vi "RSZVB Configure Calibration Standard.vi"(0 "VISA session":refnum<visa-resource-name>, 1 "Max. Freq [Hz]":dbl format="%^.3e", 2 "Length [mm]":dbl format="%^.3e", 3 "Loss":dbl format="%^.3e", 4 "C0/L0 (0.0)":dbl format="%^.3e", 5 "C1/L1 (0.0)":dbl format="%^.3e", 7 "error in (no error)":errorcluster {"code" format="%.0x"}, 8 "Min. Freq [Hz]":dbl format="%^.3e", 9 "C2/L2 (0.0)":dbl format="%^.3e", 10 "Serial Number":string, 12 "Kit":string, 13 "C3/L3 (0.0)":dbl format="%^.3e", 14 "Standard (0: Through (MM))":u16(ring) items=["Through (MM)", "Through (FF)", "Through (MF)", "Line 1 (MM)", "Line 1 (FF)", "Line 1 (MF)", "Offset short (sexless)", "Offset short (M)", "Offset short (F)", "Attenuation (MM)", "Attenuation (FF)", "Attenuation (MF)", "Symm Network (MM)", "Symm Network (FF)", "Symm Network (MF)", "Open (M)", "Open (F)", "Short (M)", "Short (F)", "Reflect (M)", "Reflect (F)", "Match (M)", "Match (F)", "Sliding Match (M)", "Sliding Match (F)", "Line 2 (MM)", "Line 2 (FF)", "Line 2 (MF)", "Line 3 (MM)", "Line 3 (FF)", "Line 3 (MF)", "Offset short 2 (M)", "Offset short 2 (F)", "Offset short 3 (M)", "Offset short 3 (F)"], 16 "Connector Type (0: N 50 ohms Kit)":i32(ring) items=["N 50 ohms Kit", "N 75 ohms Kit", "SMA Kit", "PC 7 Kit", "PC 3.5 Kit", "Sexless Usr Conn 1", "Usr Conn 2", "2.92mm Kit"], 17 "Approximation (0: Open)":i32(ring) items=["Open", "Short"]) -> (20 "dup VISA session":refnum<visa-resource-name>, 27 "error out":errorcluster {"code" format="%.0x"})   [LabVIEW 2011]
doc: "This VI defines the parameters of a calibration standard <std_type> for a specified connector type <conn_type>. A particular physical standard can be selected by specifying the name of the calibration kit and its serial number.\n\nRemote-control command(s):\n[SENSe<Ch>:]CORRection:CKIT:<conn_type>:<std_type> '<Ckit_Name>','<Std_No>',<Min_Freq>,<Max_Freq>,<El_Length>,<Loss>,<C0> | <L0>,<C1> | <L1>,<C2> | <L2>,<C3> | <L3>, OPEN | SHORt"
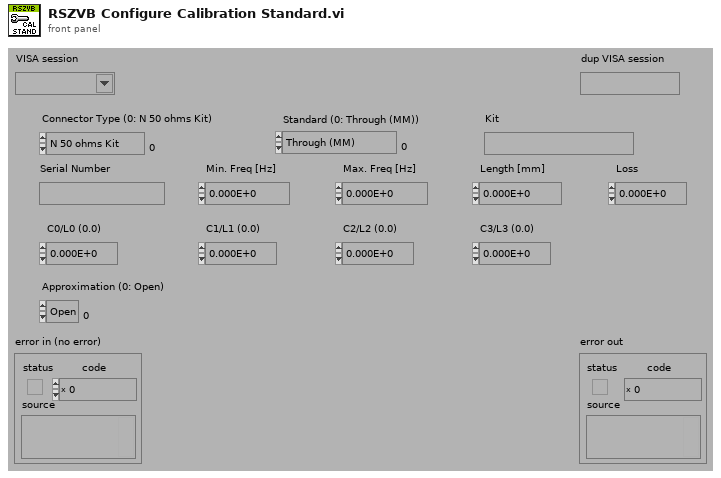
[diagram p1: front panel]
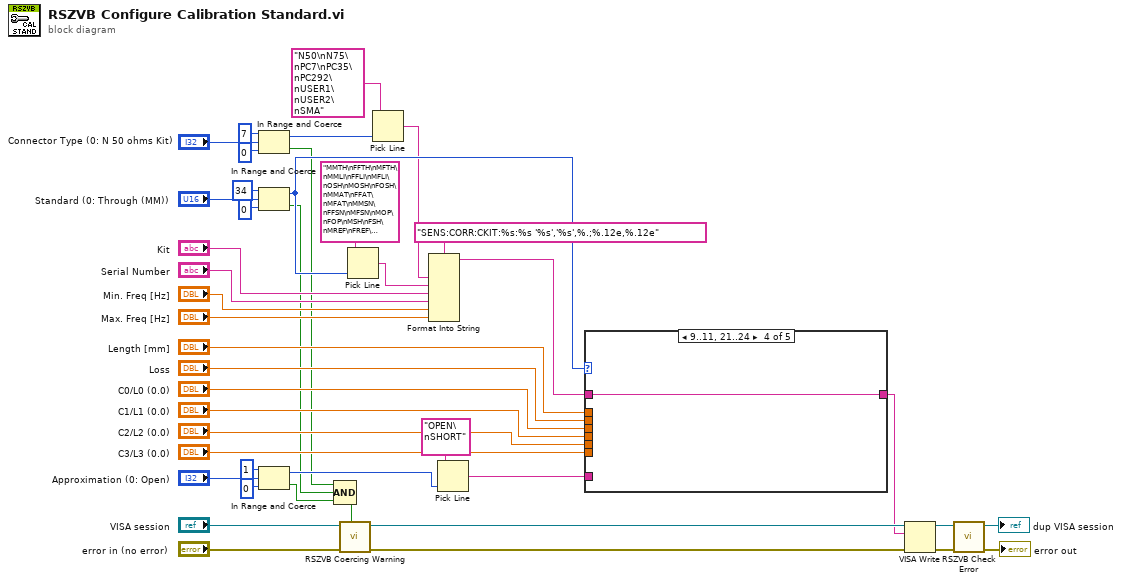
[diagram p0: block diagram]
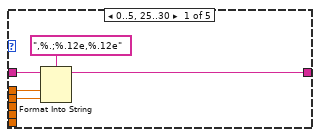
[diagram p2: hidden frame]
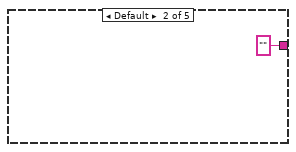
[diagram p3: hidden frame]
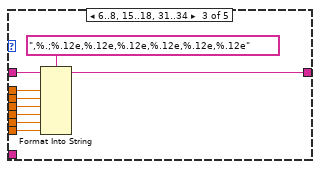
[diagram p4: hidden frame]
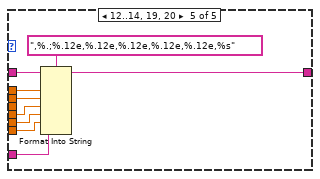
[diagram p5: hidden frame]
diagram:
  n1 = In Range and Coerce(upper limit=7 ("lower limit"), x="Connector Type (0: N 50 ohms Kit)", lower limit=0) -> (coerced(x)=w27:i32, In Range?=w2:bool)
  n2 = In Range and Coerce(upper limit=u16 34 ("lower limit"), x="Standard (0: Through (MM))", lower limit=u16 0) -> (coerced(x)=w13:u16, In Range?=w3:bool)
  n3 = In Range and Coerce(upper limit=1 ("lower limit"), x="Approximation (0: Open)", lower limit=0) -> (coerced(x)=w4:i32, In Range?=w18:bool)
  n4 = Compound Arithmetic op=AND(w2, w3, w18) -> (w17:bool)
  n5 = call "RSZVB Coercing Warning.vi"("In Range?"=w17, "error in (no error)"="error in (no error)", "VISA session"="VISA session") -> ("error out"=w42:errorcluster, "dup VISA session"=w43:refnum<visa-resource-name>)  [unwired: 7 in]
  n6 = Pick Line(multi-line string="MMTH\nFFTH\nMFTH\nMMLI\nFFLI\nMFLI\nOSH\nMOSH\nFOSH\nMMAT\nFFAT\nMFAT\nMMSN\nFFSN\nMFSN\nMOP\nFOP\nMSH\nFSH\nMREF\nFREF\nMMTC\nFMTC\nMSM\nFSM\nMMLI2\nFFLI2\nMFLI2\nMMLI3\nFFLI3\nMFLI3\nMOSHORT2\nFOSHORT2\nMOSHORT3\nFOSHORT3", line index=w13) -> (output string=w7:string)  [unwired: 1 in]
  n7 = Pick Line(multi-line string="N50\nN75\nPC7\nPC35\nPC292\nUSER1\nUSER2\nSMA", line index=w27) -> (output string=w6:string)  [unwired: 1 in]
  n8 = Format Into String(format string="SENS:CORR:CKIT:%s:%s '%s','%s',%.;%.12e,%.12e", w6, w7, "Kit", "Serial Number", "Min. Freq [Hz]", "Max. Freq [Hz]") -> (resulting string=w5:string)  [unwired: 2 in, 1 out]
  n9 = Pick Line(multi-line string="OPEN\nSHORT", line index=w4) -> (output string=w19:string)  [unwired: 1 in]
  n10 = case shown="9..11, 21..24" w13 {
    tunnel: "Length [mm]" -> [w46 _ w57 _ w67]
    tunnel: "Loss" -> [w45 _ w56 _ w66]
    tunnel: "C0/L0 (0.0)" -> [_ _ w55 _ _]
    tunnel: "C1/L1 (0.0)" -> [_ _ w54 _ w65]
    tunnel: "C2/L2 (0.0)" -> [_ _ w53 _ w64]
    tunnel: "C3/L3 (0.0)" -> [_ _ w52 _ w63]
    tunnel: w19 -> [_ _ _ _ w62]
    tunnel: w5 -> [w47 _ w50 w59 w61]
    tunnel: [w44 "" w51 w59 w60] -> w1
    frame 0..5, 25..30 {
      n11 = Format Into String(format string=",%.;%.12e,%.12e", initial string=w47, w46, w45) -> (resulting string=w44:string)  [unwired: 1 in, 1 out]
    }
    frame Default {
      (unwired) ""
    }
    frame 6..8, 15..18, 31..34 {
      n12 = Format Into String(format string=",%.;%.12e,%.12e,%.12e,%.12e,%.12e,%.12e", initial string=w50, w57, w56, w55, w54, w53, w52) -> (resulting string=w51:string)  [unwired: 1 in, 1 out]
    }
    frame 9..11, 21..24 {
    }
    frame 12..14, 19, 20 {
      n13 = Format Into String(format string=",%.;%.12e,%.12e,%.12e,%.12e,%.12e,%s", initial string=w61, w67, w66, w65, w64, w63, w62) -> (resulting string=w60:string)  [unwired: 1 in, 1 out]
    }
  }
  n14 = VISA Write(VISA resource name=w43, write buffer=w1, error in (no error)=w42) -> (VISA resource name out=w40:refnum<visa-resource-name>, error out=w41:errorcluster)  [unwired: 1 out]
  n15 = call "RSZVB Check Error.vi"("error in (no error)"=w41, "VISA session"=w40) -> ("error out"=→"error out":errorcluster, "dup VISA session"=→"dup VISA session":refnum<visa-resource-name>)  [unwired: 8 in]
